vi "Motor Controller Change RPM gracefully.vi"(0 "COM port":refnum<visa-resource-name>, 5 "RS-485 addr.":u8, 7 "RPM setpoint":sgl, 9 "Settling time (ms)":u32=20000, 11 "Close port after action":bool) -> (4 "COM port out":refnum<visa-resource-name>, 15 "Error out":errorcluster)   [LabVIEW 2020]
uses:
  ctls/CTRL_Cmd.ctl
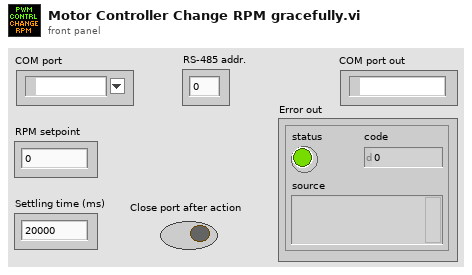
[diagram p1: front panel]
types:
  T1 = typedef "CTRL_Cmd.ctl" = string
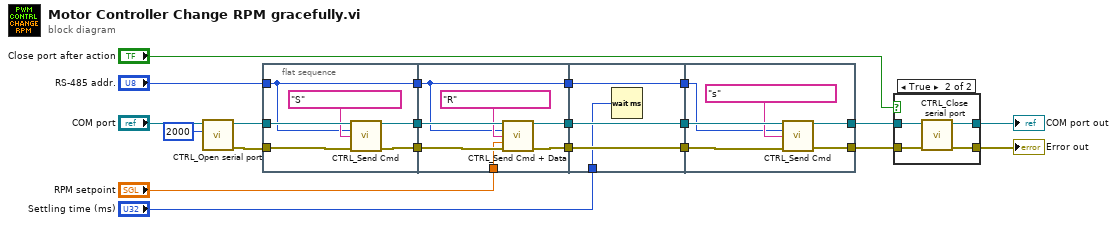
[diagram p0: block diagram]
diagram:
  n1 = call "CTRL_Open serial port.vi"("timeout (ms)"=u32 2000, "VISA resource name"="COM port") -> ("Error out"=w18:errorcluster, "VISA resource name out"=w19:refnum<visa-resource-name>)  [unwired: 8 in]
  n2 = flat-sequence {
    tunnel: w18 -> [w26]
    tunnel: w19 -> [w27]
    tunnel: [w25] -> w7
    tunnel: [w24] -> w6
    tunnel: "RS-485 addr." -> [w22]
    tunnel: [w22] -> w4
    tunnel: "RPM setpoint" -> [w32]
    tunnel: [w31] -> w11
    tunnel: [w30] -> w10
    tunnel: w7 -> [w34]
    tunnel: w6 -> [w33]
    tunnel: w4 -> [w28]
    tunnel: [w28] -> w2
    tunnel: w11 -> [w38]
    tunnel: w10 -> [w37]
    tunnel: [w38] -> w9
    tunnel: [w37] -> w8
    tunnel: [w36] -> w3
    tunnel: w2 -> [w36]
    tunnel: "Settling time (ms)" -> [w35]
    tunnel: [w41] -> w15
    tunnel: [w43] -> w16
    tunnel: w9 -> [w44]
    tunnel: w8 -> [w42]
    tunnel: w3 -> [w39]
    frame #0 {
      n3 = call "CTRL_Send Cmd.vi"("Port"=w27, "RS-485 addr."=w22, "Cmd"=T1 "S", "Error In"=w26) -> ("Port out"=w25:refnum<visa-resource-name>, "Error Out"=w24:errorcluster)  [unwired: 10 in]
    }
    frame #1 {
      n4 = call "CTRL_Send Cmd + Data.vi"("Port"=w34, "RS-485 addr."=w28, "Cmd"=T1 "R", "Data"=w32, "Error In"=w33) -> ("Port out"=w30:refnum<visa-resource-name>, "Error Out"=w31:errorcluster)  [unwired: 9 in]
    }
    frame #2 {
      n5 = Wait (ms)(milliseconds to wait=w35) -> ()  [unwired: 1 out]
    }
    frame #3 {
      n6 = call "CTRL_Send Cmd.vi"("Port"=w42, "RS-485 addr."=w39, "Cmd"=T1 "s", "Error In"=w44) -> ("Port out"=w41:refnum<visa-resource-name>, "Error Out"=w43:errorcluster)  [unwired: 10 in]
    }
  }
  n7 = case shown="True" "Close port after action" {
    tunnel: [w46 w49] -> w14
    tunnel: w15 -> [w45 w47]
    tunnel: w16 -> [w46 w48]
    tunnel: [w45 w47] -> w12
    frame False {
    }
    frame True {
      n8 = call "CTRL_Close serial port.vi"("Error in"=w48, "VISA resource name"=w47) -> ("Error out"=w49:errorcluster)  [unwired: 9 in]
    }
  }
  "Error out" <- w14
  "COM port out" <- w12
